vi "未命名 1.vi"() -> ()   [LabVIEW 2012]
panel:
  out "频率":dbl
  out "峰峰值":dbl
  in  "幅值":dbl(knob)=0.001 min=0.001 max=1.0 step=0.001 scale=0.0..1.0
  out "波形图":dynamicdata(graph)
  in  "频率":i32(knob)=2 min=2 max=100 step=1 scale=0.0..100.0
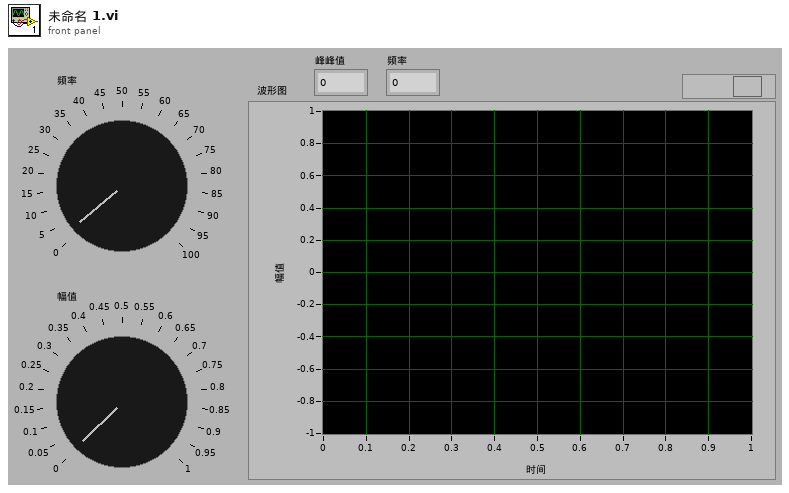
[diagram p1: front panel]
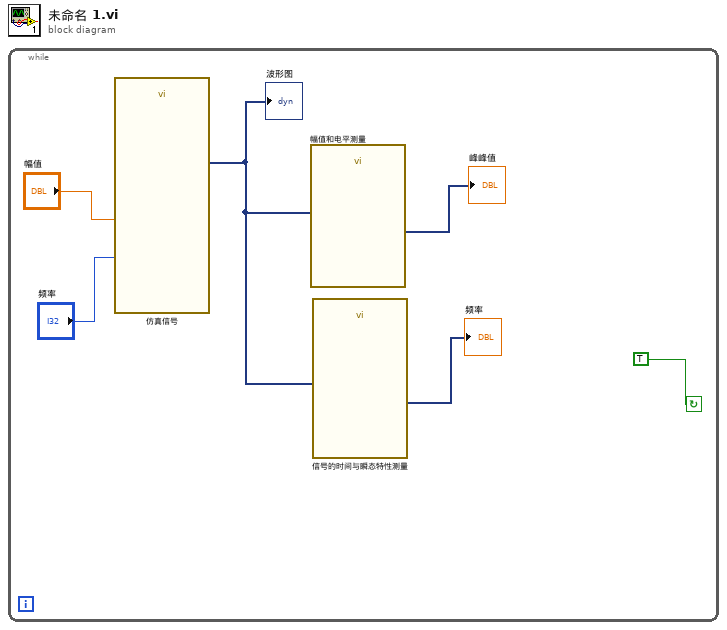
[diagram p0: block diagram]
diagram:
  n1 = while {
    stop <- TRUE continue-if-true
    n2 = call "仿真信号"("Frequency"="频率", "Amplitude"="幅值") -> ("正弦"=w3:dynamicdata)  [unwired: 4 in, 9 out]
    "波形图" <- w3
    n3 = call "幅值和电平测量"("Signals"=w3) -> ("Peak to Peak"=→"峰峰值":dynamicdata)  [unwired: 1 in, 13 out]
    n4 = call "信号的时间与瞬态特性测量"("Signals"=w3) -> ("Frequency"=→"频率":dynamicdata)  [unwired: 1 in, 9 out]
  }
